vi "Robot System.vi"(11 "Output Cluster in":T1) -> ()   [LabVIEW 2015]
uses:
  Joytsick/Controls to Cmmnds Output Clust.ctl
  Joytsick/Controls to Cmmnds Type.ctl
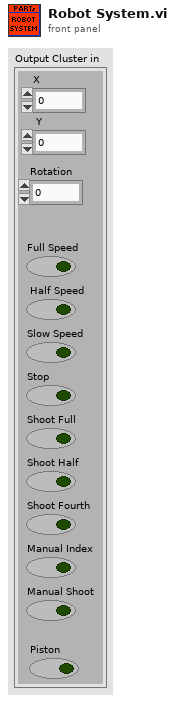
[diagram p1: front panel]
types:
  T1 = typedef "Controls to Cmmnds Output Clust.ctl" = cluster{"X ":dbl, " Y":dbl, "Rotation":dbl, "Full Speed":bool, " Half Speed":bool, "Slow Speed":bool, "Stop":bool, "Shoot Full":bool, "Shoot Half":bool, "Shoot Fourth":bool, "Manual Index":bool, "Manual Shoot":T2, "Piston":T2}
  T2 = typedef "Controls to Cmmnds Type.ctl" = bool
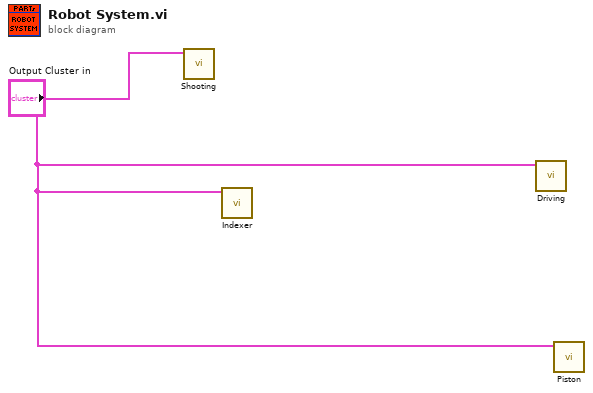
[diagram p0: block diagram]
diagram:
  n1 = call "Shooting.vi"("Output Cluster in"="Output Cluster in") -> ()  [unwired: 11 in]
  n2 = call "Indexer.vi"("Output Cluster in"="Output Cluster in") -> ()  [unwired: 11 in]
  n3 = call "Driving.vi"("Output Cluster in"="Output Cluster in") -> ()  [unwired: 11 in]
  n4 = call "Piston.vi"("Output Cluster in"="Output Cluster in") -> ()  [unwired: 11 in]
